vi "Get Display String.vi"(11 "Str Ends With in":refnum<class "Str Ends With.lvclass">) -> (2 "Display String":string)   [LabVIEW 2018, in "Str Ends With.lvclass"]
uses:
  Str Ends With.lvclass
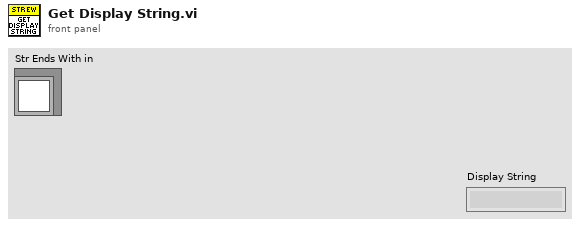
[diagram p1: front panel]
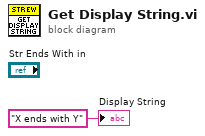
[diagram p0: block diagram]
diagram:
  "Display String" <- "X ends with Y" ("Display String")
